vi "DataTransmit.vi"(0 "数据输入":u8[](array[numeric])=array[16384 elements]) -> (2 "输出簇ADC":T4, 4 "输出簇A":T3, 5 "输出簇B":T2, 6 "总输出簇":T1, 7 "总数组":dbl[][](array[numeric]))   [LabVIEW 2014]
uses:
  DataType.ctl
panel:
  out "GlobalAMPValueFPGA":dbl
  out "GlobalAMPValueFPGAB":dbl
  out "GlobalAMPFittingBH2":dbl
  out "GlobalAMPFittingBH1":dbl
  out "GlobalAMPFittingB":dbl
  out "GlobalAMPFittingH2":dbl
  out "GlobalAMPFittingH1":dbl
  out "GlobalAMPFitting":dbl
  out "计数值":u8
  out "AD4":dbl[](array[numeric])
  out "AD3":dbl[](array[numeric])
  out "AD2":dbl[](array[numeric])
  out "AD1":dbl[](array[numeric])
  out "Yh2B":dbl[](array[numeric])
  out "Xh2B":dbl[](array[numeric])
  out "Yh1B":dbl[](array[numeric])
  out "Xh1B":dbl[](array[numeric])
  out "NoiseB":dbl[](array[numeric])
  out "FrequencyB":dbl[](array[numeric])
  out "YB":dbl[](array[numeric])
  out "XB":dbl[](array[numeric])
  out "Yh2A":dbl[](array[numeric])
  out "Xh2A":dbl[](array[numeric])
  out "Yh1A":dbl[](array[numeric])
  out "Xh1A":dbl[](array[numeric])
  out "NoiseA":dbl[](array[numeric])
  out "FrequencyA":dbl[](array[numeric])
  out "YA":dbl[](array[numeric])
  out "XA":dbl[](array[numeric])
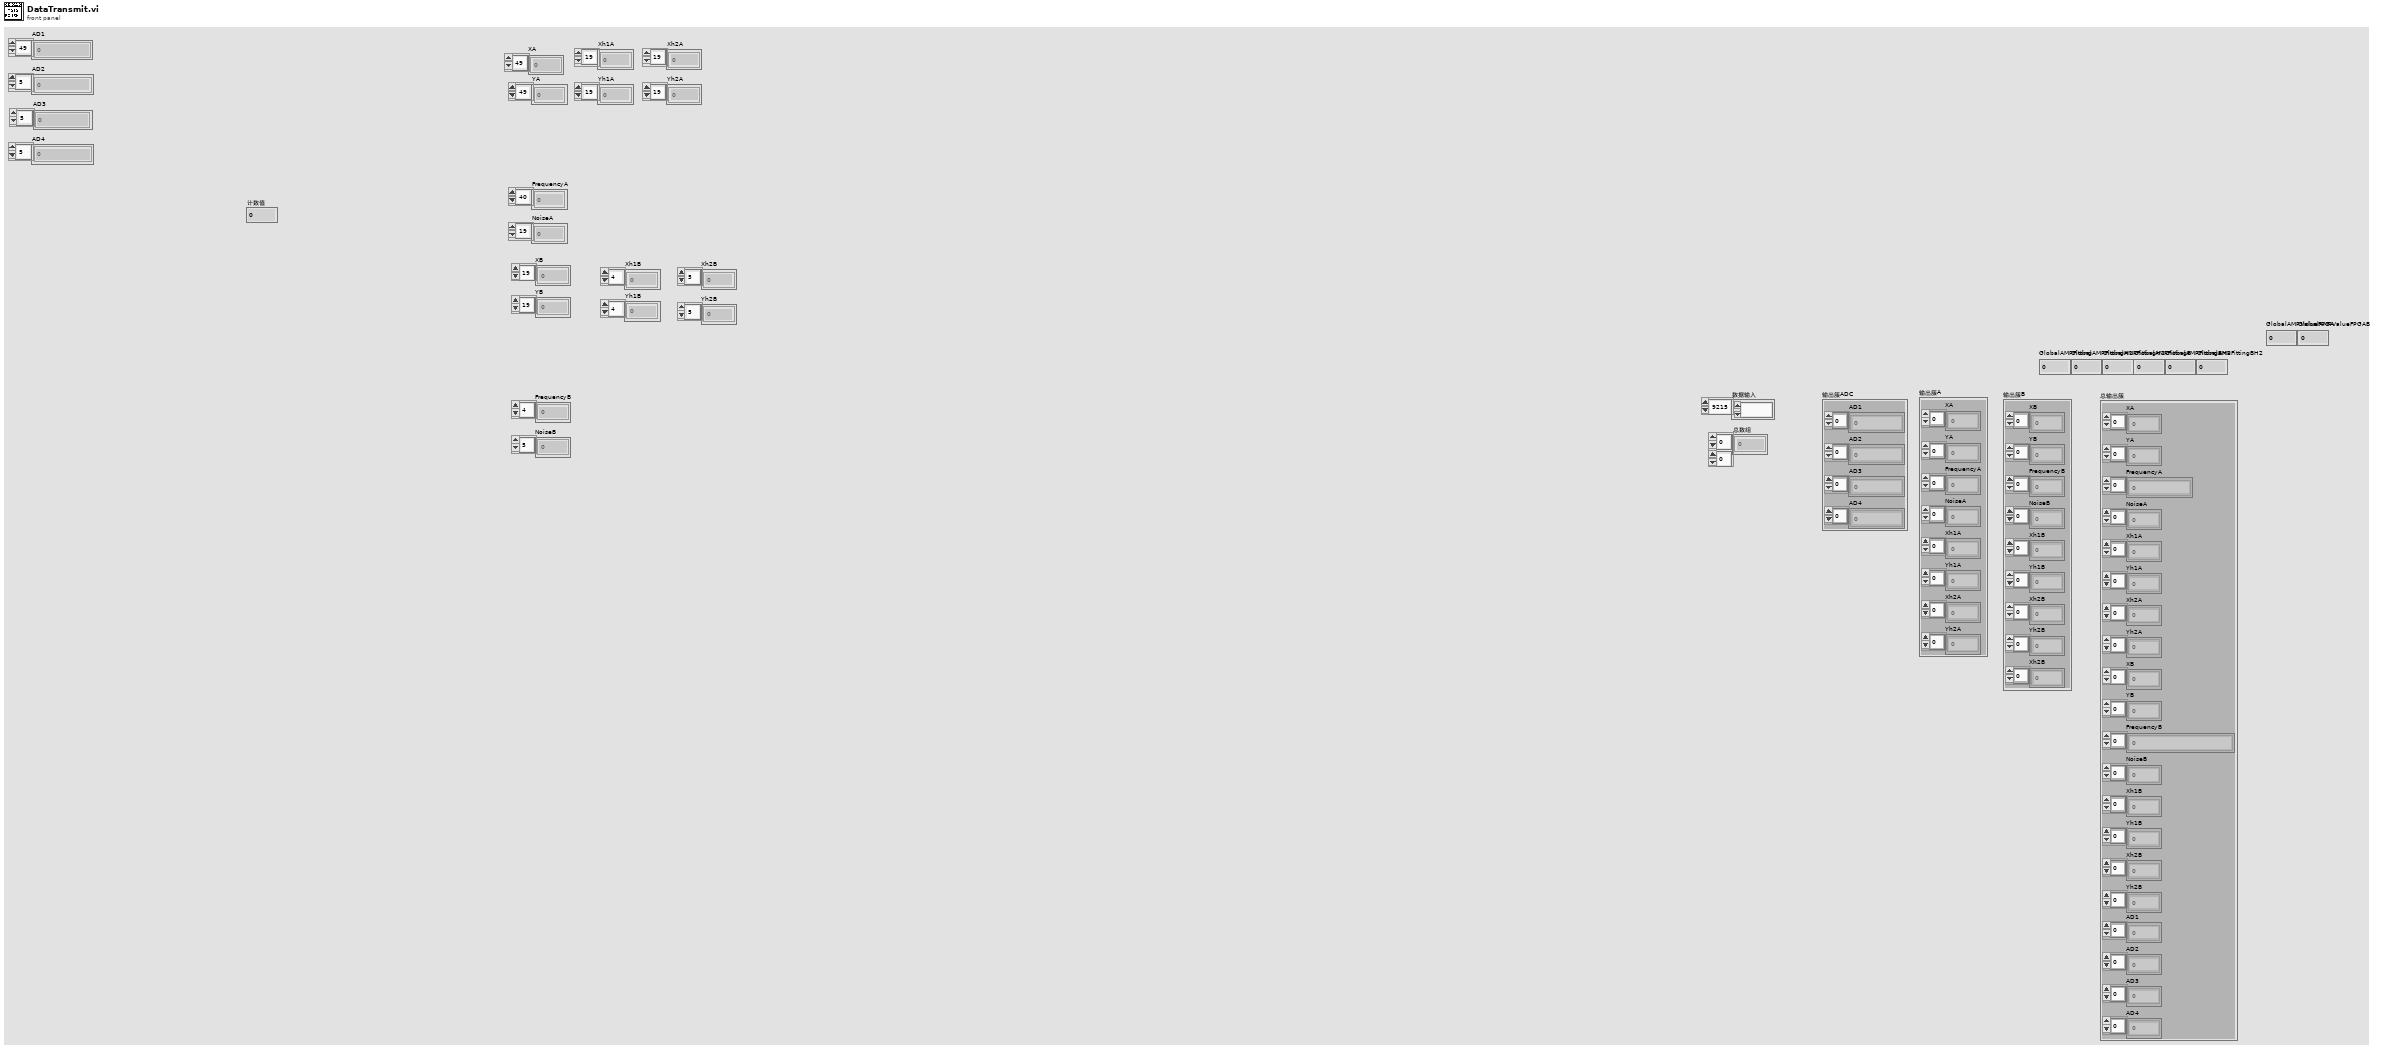
[diagram p1: front panel]
types:
  T1 = cluster{"XA":dbl[], "YA":dbl[], "FrequencyA":dbl[], "NoiseA":dbl[], "Xh1A":dbl[], "Yh1A":dbl[], "Xh2A":dbl[], "Yh2A":dbl[], "XB":dbl[], "YB":dbl[], "FrequencyB":dbl[], "NoiseB":dbl[], "Xh1B":dbl[], "Yh1B":dbl[], "Xh2B":dbl[], "Yh2B":dbl[], "AD1":dbl[], "AD2":dbl[], "AD3":dbl[], "AD4":dbl[]}
  T2 = cluster{"XB":dbl[], "YB":dbl[], "FrequencyB":dbl[], "NoiseB":dbl[], "Xh1B":dbl[], "Yh1B":dbl[], "Xh2B":dbl[], "Yh2B":dbl[], "Xh2B":dbl[]}
  T3 = cluster{"XA":dbl[], "YA":dbl[], "FrequencyA":dbl[], "NoiseA":dbl[], "Xh1A":dbl[], "Yh1A":dbl[], "Xh2A":dbl[], "Yh2A":dbl[]}
  T4 = cluster{"AD1":dbl[], "AD2":dbl[], "AD3":dbl[], "AD4":dbl[]}
  T5 = typedef "DataType.ctl" = u16
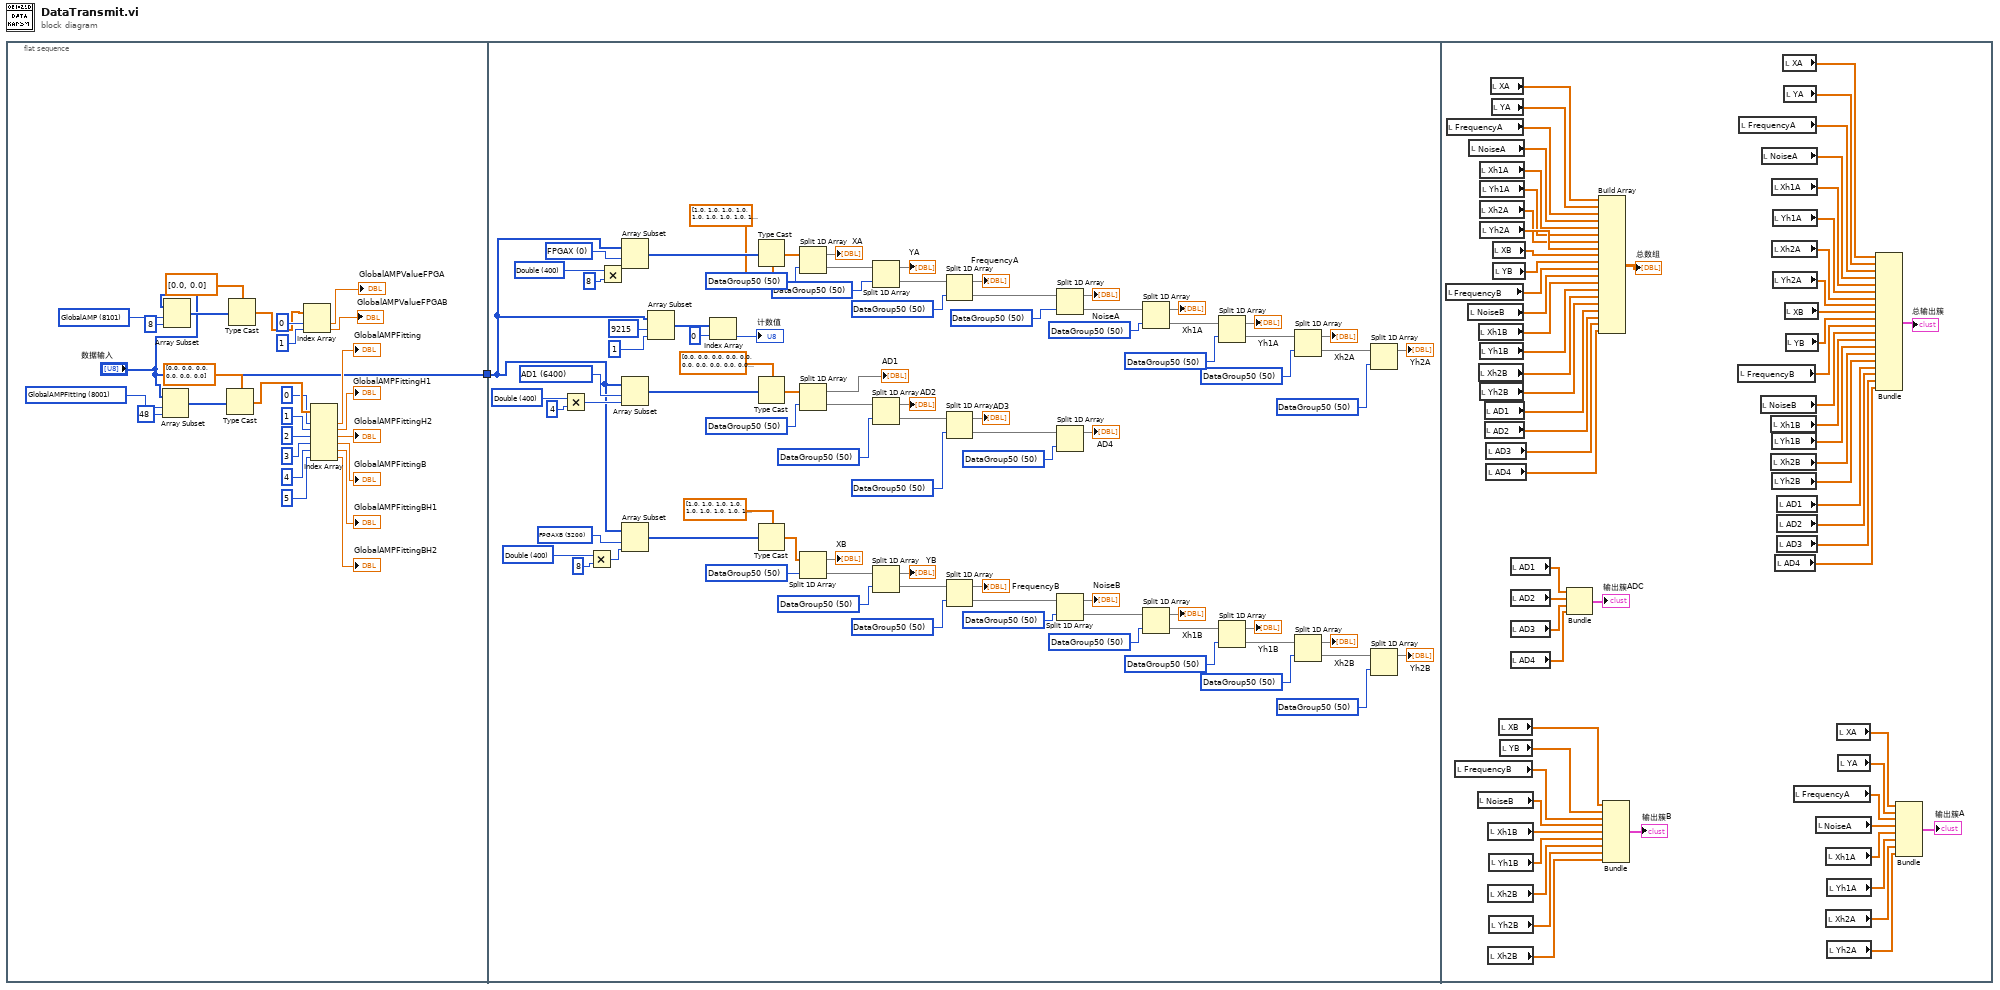
[diagram p0: block diagram]
diagram:
  n1 = flat-sequence {
    tunnel: ["数据输入"] -> w1
    tunnel: w1 -> [w29]
    frame #0 {
      w8 = u32 8101 items=["FPGAX"=0, "FPGAY"=400, "FPGAFreq"=800, "FPGANOISE"=1200, "FPGAXHARM1"=1600, "FPGAYHARM1"=2000, "FPGAXHARM2  "=2400, "FPGAYHARM2  "=2800, "FPGAXB"=3200, "FPGAYB"=3600, "FPGAFreqB"=4000, "FPGANOISEB"=4400, "FPGAXHARM1B"=4800, "FPGAYHARM1B"=5200, "FPGAXHARM2B "=5600, "FPGAYHARM2B "=6000, "AD1           "=6400, "AD2           "=6800, "AD3           "=7200, "AD4   "=7600, "GlobalAMPFitting"=8001, "GlobalAMP"=8101, "FPGAFreq"=7455, "InternalFreqvalue"=7463, "GlobalRefPhaseSlope"=7471, "HarmValue1"=7472, "HarmValue2"=7480, "REFReserve"=7488, "GlobalSweepType"=7496, "InternalSweepSartFreqvalue"=7497, "InternalSweepStopFreqvalue"=7505, "InternalSweepStepFreqvalue"=7513, "InternalSweepStepPercentValue"=7521, "InternalSweepTimeValue"=7525, "GlobalSweepTrigger"=7533, "INTReserve"=7534, "SineOutFixedVoltageValue"=7542, "GlobalSineOutSweepType"=7546, "SineOutSweepStartValue"=7547, "SineOutSweepStopValue"=7551, "SineOutSweepStepValue"=7555, "SineOutSweepStepPercentValue"=7559, "SineOutSweepTimeValue"=7563, "GlobalSineOutSweepTrigger"=7571, "SineReserve"=7572, "EquationC1"=7580, "EquationC2"=7588, "GlobalEquationTypeA"=7596, "GlobalEquationTypeB"=7601, "GlobalEquationTypeC"=7604, "EquatReserve"=7608, "GlobalGainTCSensitivity"=7640, "GlobalGainTCReserve"=7641, "GlobalInputFilterSource"=7642, "GlobalInputFilterGrounding"=7643, "GlobalInputFilterCoupling"=7644, "GlobalInputFilterNotches"=7645, "InputReserve"=7646, "GlobalGainTCTimeConstant"=7654, "GlobalGainTCFliter"=7655, "GlobalGainTCSynchronous"=7656, "FliterReserve"=7657, "GlobalOutputCH1Source"=7665, "GlobalOutputCH2Source"=7666, "Offsetvalue"=7667, "Expandvalue"=7671, "GlobalOutputSpeed"=7673, "GlobalOutputSpeedCH2"=7674, "ChannelReserve"=7675, "SampleStepTimeValue"=7691, "SampleLengthValue"=7699, "Buffer1Source"=7707, "Buffer2Source"=7708, "Buffer3Source"=7709, "Buffer4Source"=7710, "GlobalSampleTriggerMode"=7711, "GlobalSampleRunMode"=7712, "SampleCurrentPoints"=7713, "SampleReserve"=7721, "InputOvldStatusflag"=7729, "GainOvldStatusflag"=7730, "FPGAFreqShift"=7731, "SystemReserve"=7732, "GlobalRefPhasePhaseB"=7800, "GlobalRefPhaseSourceB"=7804, "FPGAFreqB"=7805, "InternalFreqvalueB"=7813, "GlobalRefPhaseSlopeB"=7821, "HarmValue1B"=7822, "HarmValue2B"=7830, "REFReserveB"=7838, "GlobalSweepTypeB"=7846, "InternalSweepSartFreqvalueB"=7847, "InternalSweepStopFreqvalueB"=7855, "InternalSweepStepFreqvalueB"=7863, "InternalSweepStepPercentValueB"=7871, "InternalSweepTimeValueB"=7875, "GlobalSweepTriggerB"=7883, "INTReserveB"=7884, "SineOutFixedVoltageValueB"=7892, "GlobalSineOutSweepTypeB"=7896, "SineOutSweepStartValueB"=7897, "SineOutSweepStopValueB"=7901, "SineOutSweepStepValueB"=7905, "SineOutSweepStepPercentValueB"=7909, "SineOutSweepTimeValueB"=7913, "GlobalSineOutSweepTriggerB"=7921, "SineReserveB"=7922, "EquationC1B"=7930, "EquationC2B"=7938, "GlobalEquationTypeAB"=7946, "GlobalEquationTypeBB"=7950, "GlobalEquationTypeCB"=7954, "EquatReserveB"=7958, "GlobalGainTCSensitivityB"=7990, "GlobalGainTCReserveB"=7991, "GlobalInputFilterSourceB"=7992, "GlobalInputFilterGroundingB"=7993, "GlobalInputFilterCouplingB"=7994, "GlobalInputFilterNotchesB"=7995, "InputReserveB"=7996, "GlobalGainTCTimeConstantB"=8004, "GlobalGainTCFliterB"=8005, "GlobalGainTCSynchronousB"=8006, "FliterReserveB"=8007, "GlobalOutputCH1Source"=8015, "GlobalOutputCH2Source"=8016, "OffsetvalueB"=8017, "ExpandvalueB"=8021, "GlobalOutputSpeedB"=8023, "GlobalOutputSpeedCH2B"=8024, "ChannelReserve"=8025, "SampleStepTimeValueB"=8041, "SampleLengthValueB"=8049, "Buffer1SourceB"=8057, "Buffer2SourceB"=8058, "Buffer3SourceB"=8059, "Buffer4SourceB"=8060, "GlobalSampleTriggerModeB"=8061, "GlobalSampleRunModeB"=8062, "SampleCurrentPointsB"=8063, "SampleReserveB"=8071, "InputOvldStatusflagB"=8079, "GainOvldStatusflagB"=8080, "FPGAFreqShiftB"=8081, "SystemReserveB"=8082] ("下拉列表")
      w28 = u32 8001 items=["FPGAX"=0, "FPGAY"=400, "FPGAFreq"=800, "FPGANOISE"=1200, "FPGAXHARM1"=1600, "FPGAYHARM1"=2000, "FPGAXHARM2  "=2400, "FPGAYHARM2  "=2800, "FPGAXB"=3200, "FPGAYB"=3600, "FPGAFreqB"=4000, "FPGANOISEB"=4400, "FPGAXHARM1B"=4800, "FPGAYHARM1B"=5200, "FPGAXHARM2B "=5600, "FPGAYHARM2B "=6000, "AD1           "=6400, "AD2           "=6800, "AD3           "=7200, "AD4   "=7600, "GlobalAMPFitting"=8001, "GlobalAMP"=8101, "FPGAFreq"=7455, "InternalFreqvalue"=7463, "GlobalRefPhaseSlope"=7471, "HarmValue1"=7472, "HarmValue2"=7480, "REFReserve"=7488, "GlobalSweepType"=7496, "InternalSweepSartFreqvalue"=7497, "InternalSweepStopFreqvalue"=7505, "InternalSweepStepFreqvalue"=7513, "InternalSweepStepPercentValue"=7521, "InternalSweepTimeValue"=7525, "GlobalSweepTrigger"=7533, "INTReserve"=7534, "SineOutFixedVoltageValue"=7542, "GlobalSineOutSweepType"=7546, "SineOutSweepStartValue"=7547, "SineOutSweepStopValue"=7551, "SineOutSweepStepValue"=7555, "SineOutSweepStepPercentValue"=7559, "SineOutSweepTimeValue"=7563, "GlobalSineOutSweepTrigger"=7571, "SineReserve"=7572, "EquationC1"=7580, "EquationC2"=7588, "GlobalEquationTypeA"=7596, "GlobalEquationTypeB"=7601, "GlobalEquationTypeC"=7604, "EquatReserve"=7608, "GlobalGainTCSensitivity"=7640, "GlobalGainTCReserve"=7641, "GlobalInputFilterSource"=7642, "GlobalInputFilterGrounding"=7643, "GlobalInputFilterCoupling"=7644, "GlobalInputFilterNotches"=7645, "InputReserve"=7646, "GlobalGainTCTimeConstant"=7654, "GlobalGainTCFliter"=7655, "GlobalGainTCSynchronous"=7656, "FliterReserve"=7657, "GlobalOutputCH1Source"=7665, "GlobalOutputCH2Source"=7666, "Offsetvalue"=7667, "Expandvalue"=7671, "GlobalOutputSpeed"=7673, "GlobalOutputSpeedCH2"=7674, "ChannelReserve"=7675, "SampleStepTimeValue"=7691, "SampleLengthValue"=7699, "Buffer1Source"=7707, "Buffer2Source"=7708, "Buffer3Source"=7709, "Buffer4Source"=7710, "GlobalSampleTriggerMode"=7711, "GlobalSampleRunMode"=7712, "SampleCurrentPoints"=7713, "SampleReserve"=7721, "InputOvldStatusflag"=7729, "GainOvldStatusflag"=7730, "FPGAFreqShift"=7731, "SystemReserve"=7732, "GlobalRefPhasePhaseB"=7800, "GlobalRefPhaseSourceB"=7804, "FPGAFreqB"=7805, "InternalFreqvalueB"=7813, "GlobalRefPhaseSlopeB"=7821, "HarmValue1B"=7822, "HarmValue2B"=7830, "REFReserveB"=7838, "GlobalSweepTypeB"=7846, "InternalSweepSartFreqvalueB"=7847, "InternalSweepStopFreqvalueB"=7855, "InternalSweepStepFreqvalueB"=7863, "InternalSweepStepPercentValueB"=7871, "InternalSweepTimeValueB"=7875, "GlobalSweepTriggerB"=7883, "INTReserveB"=7884, "SineOutFixedVoltageValueB"=7892, "GlobalSineOutSweepTypeB"=7896, "SineOutSweepStartValueB"=7897, "SineOutSweepStopValueB"=7901, "SineOutSweepStepValueB"=7905, "SineOutSweepStepPercentValueB"=7909, "SineOutSweepTimeValueB"=7913, "GlobalSineOutSweepTriggerB"=7921, "SineReserveB"=7922, "EquationC1B"=7930, "EquationC2B"=7938, "GlobalEquationTypeAB"=7946, "GlobalEquationTypeBB"=7950, "GlobalEquationTypeCB"=7954, "EquatReserveB"=7958, "GlobalGainTCSensitivityB"=7990, "GlobalGainTCReserveB"=7991, "GlobalInputFilterSourceB"=7992, "GlobalInputFilterGroundingB"=7993, "GlobalInputFilterCouplingB"=7994, "GlobalInputFilterNotchesB"=7995, "InputReserveB"=7996, "GlobalGainTCTimeConstantB"=8004, "GlobalGainTCFliterB"=8005, "GlobalGainTCSynchronousB"=8006, "FliterReserveB"=8007, "GlobalOutputCH1Source"=8015, "GlobalOutputCH2Source"=8016, "OffsetvalueB"=8017, "ExpandvalueB"=8021, "GlobalOutputSpeedB"=8023, "GlobalOutputSpeedCH2B"=8024, "ChannelReserve"=8025, "SampleStepTimeValueB"=8041, "SampleLengthValueB"=8049, "Buffer1SourceB"=8057, "Buffer2SourceB"=8058, "Buffer3SourceB"=8059, "Buffer4SourceB"=8060, "GlobalSampleTriggerModeB"=8061, "GlobalSampleRunModeB"=8062, "SampleCurrentPointsB"=8063, "SampleReserveB"=8071, "InputOvldStatusflagB"=8079, "GainOvldStatusflagB"=8080, "FPGAFreqShiftB"=8081, "SystemReserveB"=8082] ("下拉列表")
      n2 = Array Subset(array="数据输入", index=w28, length=48 ("长度")) -> (w25:u8[])
      n3 = Array Subset(array="数据输入", index=w8, length=8 ("长度")) -> (w11:u8[])
      n4 = Type Cast(type=dbl[] [0.0, 0.0, 0.0, 0.0, 0.0, 0.0], x=w25) -> (*(type *) &x=w24:dbl[])
      n5 = Type Cast(type=sgl[] [0.0, 0.0], x=w11) -> (*(type *) &x=w2:sgl[])
      n6 = Index Array(array=w2, index #1=0 ("索引"), index #2=1 ("索引 2")) -> (element #1=→"GlobalAMPValueFPGA":sgl, element #2=→"GlobalAMPValueFPGAB":sgl)
      n7 = Index Array(array=w24, index #1=0 ("索引"), index #2=1 ("索引 2"), index #3=2 ("索引 3"), index #4=3 ("索引 4"), index #5=4 ("索引 5"), index #6=5 ("索引 6")) -> (element #1=→"GlobalAMPFitting":dbl, element #2=→"GlobalAMPFittingH1":dbl, element #3=→"GlobalAMPFittingH2":dbl, element #4=→"GlobalAMPFittingB":dbl, element #5=→"GlobalAMPFittingBH1":dbl, element #6=→"GlobalAMPFittingBH2":dbl)
    }
    frame #1 {
      w112 = u16 50 items=["unsignedInt8"=1, "unsignedInt16"=2, "unsignedInt32"=4, "unsignedInt64"=8, "Float"=80, "Double"=160, "StartLength"=2240, "DataGroup50"=50, "DataGroup20"=20] ("数据类型")
      w111 = u16 50 items=["unsignedInt8"=1, "unsignedInt16"=2, "unsignedInt32"=4, "unsignedInt64"=8, "Float"=80, "Double"=160, "StartLength"=2240, "DataGroup50"=50, "DataGroup20"=20] ("数据类型")
      w109 = u16 50 items=["unsignedInt8"=1, "unsignedInt16"=2, "unsignedInt32"=4, "unsignedInt64"=8, "Float"=80, "Double"=160, "StartLength"=2240, "DataGroup50"=50, "DataGroup20"=20] ("数据类型")
      w108 = u16 50 items=["unsignedInt8"=1, "unsignedInt16"=2, "unsignedInt32"=4, "unsignedInt64"=8, "Float"=80, "Double"=160, "StartLength"=2240, "DataGroup50"=50, "DataGroup20"=20] ("数据类型")
      w107 = u16 50 items=["unsignedInt8"=1, "unsignedInt16"=2, "unsignedInt32"=4, "unsignedInt64"=8, "Float"=80, "Double"=160, "StartLength"=2240, "DataGroup50"=50, "DataGroup20"=20] ("数据类型")
      w106 = u16 50 items=["unsignedInt8"=1, "unsignedInt16"=2, "unsignedInt32"=4, "unsignedInt64"=8, "Float"=80, "Double"=160, "StartLength"=2240, "DataGroup50"=50, "DataGroup20"=20] ("数据类型")
      w105 = u16 50 items=["unsignedInt8"=1, "unsignedInt16"=2, "unsignedInt32"=4, "unsignedInt64"=8, "Float"=80, "Double"=160, "StartLength"=2240, "DataGroup50"=50, "DataGroup20"=20] ("数据类型")
      w110 = u16 50 items=["unsignedInt8"=1, "unsignedInt16"=2, "unsignedInt32"=4, "unsignedInt64"=8, "Float"=80, "Double"=160, "StartLength"=2240, "DataGroup50"=50, "DataGroup20"=20] ("数据类型")
      w104 = u16 50 items=["unsignedInt8"=1, "unsignedInt16"=2, "unsignedInt32"=4, "unsignedInt64"=8, "Float"=80, "Double"=160, "StartLength"=2240, "DataGroup50"=50, "DataGroup20"=20] ("数据类型")
      w103 = u16 50 items=["unsignedInt8"=1, "unsignedInt16"=2, "unsignedInt32"=4, "unsignedInt64"=8, "Float"=80, "Double"=160, "StartLength"=2240, "DataGroup50"=50, "DataGroup20"=20] ("数据类型")
      w96 = T5 400 items=["unsignedInt8"=1, "unsignedInt16"=2, "unsignedInt32"=4, "unsignedInt64"=8, "Float"=200, "Double"=400] ("数据类型")
      w95 = u32 3200 items=["FPGAX"=0, "FPGAY"=400, "FPGAFreq"=800, "FPGANOISE"=1200, "FPGAXHARM1"=1600, "FPGAYHARM1"=2000, "FPGAXHARM2  "=2400, "FPGAYHARM2  "=2800, "FPGAXB"=3200, "FPGAYB"=3600, "FPGAFreqB"=4000, "FPGANOISEB"=4400, "FPGAXHARM1B"=4800, "FPGAYHARM1B"=5200, "FPGAXHARM2B "=5600, "FPGAYHARM2B "=6000, "AD1           "=6400, "AD2           "=6800, "AD3           "=7200, "AD4   "=7600, "GlobalRefPhasePhase"=7450, "GlobalRefPhaseSource"=7454, "FPGAFreq"=7455, "InternalFreqvalue"=7463, "GlobalRefPhaseSlope"=7471, "HarmValue1"=7472, "HarmValue2"=7480, "REFReserve"=7488, "GlobalSweepType"=7496, "InternalSweepSartFreqvalue"=7497, "InternalSweepStopFreqvalue"=7505, "InternalSweepStepFreqvalue"=7513, "InternalSweepStepPercentValue"=7521, "InternalSweepTimeValue"=7525, "GlobalSweepTrigger"=7533, "INTReserve"=7534, "SineOutFixedVoltageValue"=7542, "GlobalSineOutSweepType"=7546, "SineOutSweepStartValue"=7547, "SineOutSweepStopValue"=7551, "SineOutSweepStepValue"=7555, "SineOutSweepStepPercentValue"=7559, "SineOutSweepTimeValue"=7563, "GlobalSineOutSweepTrigger"=7571, "SineReserve"=7572, "EquationC1"=7580, "EquationC2"=7588, "GlobalEquationTypeA"=7596, "GlobalEquationTypeB"=7601, "GlobalEquationTypeC"=7604, "EquatReserve"=7608, "GlobalGainTCSensitivity"=7640, "GlobalGainTCReserve"=7641, "GlobalInputFilterSource"=7642, "GlobalInputFilterGrounding"=7643, "GlobalInputFilterCoupling"=7644, "GlobalInputFilterNotches"=7645, "InputReserve"=7646, "GlobalGainTCTimeConstant"=7654, "GlobalGainTCFliter"=7655, "GlobalGainTCSynchronous"=7656, "FliterReserve"=7657, "GlobalOutputCH1Source"=7665, "GlobalOutputCH2Source"=7666, "Offsetvalue"=7667, "Expandvalue"=7671, "GlobalOutputSpeed"=7673, "GlobalOutputSpeedCH2"=7674, "ChannelReserve"=7675, "SampleStepTimeValue"=7691, "SampleLengthValue"=7699, "Buffer1Source"=7707, "Buffer2Source"=7708, "Buffer3Source"=7709, "Buffer4Source"=7710, "GlobalSampleTriggerMode"=7711, "GlobalSampleRunMode"=7712, "SampleCurrentPoints"=7713, "SampleReserve"=7721, "InputOvldStatusflag"=7729, "GainOvldStatusflag"=7730, "FPGAFreqShift"=7731, "SystemReserve"=7732, "GlobalRefPhasePhaseB"=7800, "GlobalRefPhaseSourceB"=7804, "FPGAFreqB"=7805, "InternalFreqvalueB"=7813, "GlobalRefPhaseSlopeB"=7821, "HarmValue1B"=7822, "HarmValue2B"=7830, "REFReserveB"=7838, "GlobalSweepTypeB"=7846, "InternalSweepSartFreqvalueB"=7847, "InternalSweepStopFreqvalueB"=7855, "InternalSweepStepFreqvalueB"=7863, "InternalSweepStepPercentValueB"=7871, "InternalSweepTimeValueB"=7875, "GlobalSweepTriggerB"=7883, "INTReserveB"=7884, "SineOutFixedVoltageValueB"=7892, "GlobalSineOutSweepTypeB"=7896, "SineOutSweepStartValueB"=7897, "SineOutSweepStopValueB"=7901, "SineOutSweepStepValueB"=7905, "SineOutSweepStepPercentValueB"=7909, "SineOutSweepTimeValueB"=7913, "GlobalSineOutSweepTriggerB"=7921, "SineReserveB"=7922, "EquationC1B"=7930, "EquationC2B"=7938, "GlobalEquationTypeAB"=7946, "GlobalEquationTypeBB"=7950, "GlobalEquationTypeCB"=7954, "EquatReserveB"=7958, "GlobalGainTCSensitivityB"=7990, "GlobalGainTCReserveB"=7991, "GlobalInputFilterSourceB"=7992, "GlobalInputFilterGroundingB"=7993, "GlobalInputFilterCouplingB"=7994, "GlobalInputFilterNotchesB"=7995, "InputReserveB"=7996, "GlobalGainTCTimeConstantB"=8004, "GlobalGainTCFliterB"=8005, "GlobalGainTCSynchronousB"=8006, "FliterReserveB"=8007, "GlobalOutputCH1Source"=8015, "GlobalOutputCH2Source"=8016, "OffsetvalueB"=8017, "ExpandvalueB"=8021, "GlobalOutputSpeedB"=8023, "GlobalOutputSpeedCH2B"=8024, "ChannelReserve"=8025, "SampleStepTimeValueB"=8041, "SampleLengthValueB"=8049, "Buffer1SourceB"=8057, "Buffer2SourceB"=8058, "Buffer3SourceB"=8059, "Buffer4SourceB"=8060, "GlobalSampleTriggerModeB"=8061, "GlobalSampleRunModeB"=8062, "SampleCurrentPointsB"=8063, "SampleReserveB"=8071, "InputOvldStatusflagB"=8079, "GainOvldStatusflagB"=8080, "FPGAFreqShiftB"=8081, "SystemReserveB"=8082] ("下拉列表")
      w94 = u16 50 items=["unsignedInt8"=1, "unsignedInt16"=2, "unsignedInt32"=4, "unsignedInt64"=8, "Float"=80, "Double"=160, "StartLength"=2240, "DataGroup50"=50, "DataGroup20"=20] ("数据类型")
      w93 = u16 50 items=["unsignedInt8"=1, "unsignedInt16"=2, "unsignedInt32"=4, "unsignedInt64"=8, "Float"=80, "Double"=160, "StartLength"=2240, "DataGroup50"=50, "DataGroup20"=20] ("数据类型")
      w92 = u16 50 items=["unsignedInt8"=1, "unsignedInt16"=2, "unsignedInt32"=4, "unsignedInt64"=8, "Float"=80, "Double"=160, "StartLength"=2240, "DataGroup50"=50, "DataGroup20"=20] ("数据类型")
      w91 = u16 50 items=["unsignedInt8"=1, "unsignedInt16"=2, "unsignedInt32"=4, "unsignedInt64"=8, "Float"=80, "Double"=160, "StartLength"=2240, "DataGroup50"=50, "DataGroup20"=20] ("数据类型")
      w88 = u16 50 items=["unsignedInt8"=1, "unsignedInt16"=2, "unsignedInt32"=4, "unsignedInt64"=8, "Float"=80, "Double"=160, "StartLength"=2240, "DataGroup50"=50, "DataGroup20"=20] ("数据类型")
      w87 = u16 50 items=["unsignedInt8"=1, "unsignedInt16"=2, "unsignedInt32"=4, "unsignedInt64"=8, "Float"=80, "Double"=160, "StartLength"=2240, "DataGroup50"=50, "DataGroup20"=20] ("数据类型")
      w84 = T5 400 items=["unsignedInt8"=1, "unsignedInt16"=2, "unsignedInt32"=4, "unsignedInt64"=8, "Float"=200, "Double"=400] ("数据类型")
      w83 = u32 0 items=["FPGAX"=0, "FPGAY"=400, "FPGAFreq"=800, "FPGANOISE"=1200, "FPGAXHARM1"=1600, "FPGAYHARM1"=2000, "FPGAXHARM2  "=2400, "FPGAYHARM2  "=2800, "FPGAXB"=3200, "FPGAYB"=3600, "FPGAFreqB"=4000, "FPGANOISEB"=4400, "FPGAXHARM1B"=4800, "FPGAYHARM1B"=5200, "FPGAXHARM2B "=5600, "FPGAYHARM2B "=6000, "AD1           "=6400, "AD2           "=6800, "AD3           "=7200, "AD4   "=7600, "GlobalRefPhasePhase"=7450, "GlobalRefPhaseSource"=7454, "FPGAFreq"=7455, "InternalFreqvalue"=7463, "GlobalRefPhaseSlope"=7471, "HarmValue1"=7472, "HarmValue2"=7480, "REFReserve"=7488, "GlobalSweepType"=7496, "InternalSweepSartFreqvalue"=7497, "InternalSweepStopFreqvalue"=7505, "InternalSweepStepFreqvalue"=7513, "InternalSweepStepPercentValue"=7521, "InternalSweepTimeValue"=7525, "GlobalSweepTrigger"=7533, "INTReserve"=7534, "SineOutFixedVoltageValue"=7542, "GlobalSineOutSweepType"=7546, "SineOutSweepStartValue"=7547, "SineOutSweepStopValue"=7551, "SineOutSweepStepValue"=7555, "SineOutSweepStepPercentValue"=7559, "SineOutSweepTimeValue"=7563, "GlobalSineOutSweepTrigger"=7571, "SineReserve"=7572, "EquationC1"=7580, "EquationC2"=7588, "GlobalEquationTypeA"=7596, "GlobalEquationTypeB"=7601, "GlobalEquationTypeC"=7604, "EquatReserve"=7608, "GlobalGainTCSensitivity"=7640, "GlobalGainTCReserve"=7641, "GlobalInputFilterSource"=7642, "GlobalInputFilterGrounding"=7643, "GlobalInputFilterCoupling"=7644, "GlobalInputFilterNotches"=7645, "InputReserve"=7646, "GlobalGainTCTimeConstant"=7654, "GlobalGainTCFliter"=7655, "GlobalGainTCSynchronous"=7656, "FliterReserve"=7657, "GlobalOutputCH1Source"=7665, "GlobalOutputCH2Source"=7666, "Offsetvalue"=7667, "Expandvalue"=7671, "GlobalOutputSpeed"=7673, "GlobalOutputSpeedCH2"=7674, "ChannelReserve"=7675, "SampleStepTimeValue"=7691, "SampleLengthValue"=7699, "Buffer1Source"=7707, "Buffer2Source"=7708, "Buffer3Source"=7709, "Buffer4Source"=7710, "GlobalSampleTriggerMode"=7711, "GlobalSampleRunMode"=7712, "SampleCurrentPoints"=7713, "SampleReserve"=7721, "InputOvldStatusflag"=7729, "GainOvldStatusflag"=7730, "FPGAFreqShift"=7731, "SystemReserve"=7732, "GlobalRefPhasePhaseB"=7800, "GlobalRefPhaseSourceB"=7804, "FPGAFreqB"=7805, "InternalFreqvalueB"=7813, "GlobalRefPhaseSlopeB"=7821, "HarmValue1B"=7822, "HarmValue2B"=7830, "REFReserveB"=7838, "GlobalSweepTypeB"=7846, "InternalSweepSartFreqvalueB"=7847, "InternalSweepStopFreqvalueB"=7855, "InternalSweepStepFreqvalueB"=7863, "InternalSweepStepPercentValueB"=7871, "InternalSweepTimeValueB"=7875, "GlobalSweepTriggerB"=7883, "INTReserveB"=7884, "SineOutFixedVoltageValueB"=7892, "GlobalSineOutSweepTypeB"=7896, "SineOutSweepStartValueB"=7897, "SineOutSweepStopValueB"=7901, "SineOutSweepStepValueB"=7905, "SineOutSweepStepPercentValueB"=7909, "SineOutSweepTimeValueB"=7913, "GlobalSineOutSweepTriggerB"=7921, "SineReserveB"=7922, "EquationC1B"=7930, "EquationC2B"=7938, "GlobalEquationTypeAB"=7946, "GlobalEquationTypeBB"=7950, "GlobalEquationTypeCB"=7954, "EquatReserveB"=7958, "GlobalGainTCSensitivityB"=7990, "GlobalGainTCReserveB"=7991, "GlobalInputFilterSourceB"=7992, "GlobalInputFilterGroundingB"=7993, "GlobalInputFilterCouplingB"=7994, "GlobalInputFilterNotchesB"=7995, "InputReserveB"=7996, "GlobalGainTCTimeConstantB"=8004, "GlobalGainTCFliterB"=8005, "GlobalGainTCSynchronousB"=8006, "FliterReserveB"=8007, "GlobalOutputCH1Source"=8015, "GlobalOutputCH2Source"=8016, "OffsetvalueB"=8017, "ExpandvalueB"=8021, "GlobalOutputSpeedB"=8023, "GlobalOutputSpeedCH2B"=8024, "ChannelReserve"=8025, "SampleStepTimeValueB"=8041, "SampleLengthValueB"=8049, "Buffer1SourceB"=8057, "Buffer2SourceB"=8058, "Buffer3SourceB"=8059, "Buffer4SourceB"=8060, "GlobalSampleTriggerModeB"=8061, "GlobalSampleRunModeB"=8062, "SampleCurrentPointsB"=8063, "SampleReserveB"=8071, "InputOvldStatusflagB"=8079, "GainOvldStatusflagB"=8080, "FPGAFreqShiftB"=8081, "SystemReserveB"=8082] ("下拉列表")
      w82 = u16 50 items=["unsignedInt8"=1, "unsignedInt16"=2, "unsignedInt32"=4, "unsignedInt64"=8, "Float"=80, "Double"=160, "StartLength"=2240, "DataGroup50"=50, "DataGroup20"=20] ("数据类型")
      w81 = u16 50 items=["unsignedInt8"=1, "unsignedInt16"=2, "unsignedInt32"=4, "unsignedInt64"=8, "Float"=80, "Double"=160, "StartLength"=2240, "DataGroup50"=50, "DataGroup20"=20] ("数据类型")
      w80 = u16 50 items=["unsignedInt8"=1, "unsignedInt16"=2, "unsignedInt32"=4, "unsignedInt64"=8, "Float"=80, "Double"=160, "StartLength"=2240, "DataGroup50"=50, "DataGroup20"=20] ("数据类型")
      w78 = u32 6400 items=["FPGAX"=0, "FPGAY"=400, "FPGAFreq"=800, "FPGANOISE"=1200, "FPGAXHARM1"=1600, "FPGAYHARM1"=2000, "FPGAXHARM2  "=2400, "FPGAYHARM2  "=2800, "FPGAXB"=3200, "FPGAYB"=3600, "FPGAFreqB"=4000, "FPGANOISEB"=4400, "FPGAXHARM1B"=4800, "FPGAYHARM1B"=5200, "FPGAXHARM2B "=5600, "FPGAYHARM2B "=6000, "AD1           "=6400, "AD2           "=6800, "AD3           "=7200, "AD4   "=7600, "GlobalRefPhasePhase"=7450, "GlobalRefPhaseSource"=7454, "FPGAFreq"=7455, "InternalFreqvalue"=7463, "GlobalRefPhaseSlope"=7471, "HarmValue1"=7472, "HarmValue2"=7480, "REFReserve"=7488, "GlobalSweepType"=7496, "InternalSweepSartFreqvalue"=7497, "InternalSweepStopFreqvalue"=7505, "InternalSweepStepFreqvalue"=7513, "InternalSweepStepPercentValue"=7521, "InternalSweepTimeValue"=7525, "GlobalSweepTrigger"=7533, "INTReserve"=7534, "SineOutFixedVoltageValue"=7542, "GlobalSineOutSweepType"=7546, "SineOutSweepStartValue"=7547, "SineOutSweepStopValue"=7551, "SineOutSweepStepValue"=7555, "SineOutSweepStepPercentValue"=7559, "SineOutSweepTimeValue"=7563, "GlobalSineOutSweepTrigger"=7571, "SineReserve"=7572, "EquationC1"=7580, "EquationC2"=7588, "GlobalEquationTypeA"=7596, "GlobalEquationTypeB"=7601, "GlobalEquationTypeC"=7604, "EquatReserve"=7608, "GlobalGainTCSensitivity"=7640, "GlobalGainTCReserve"=7641, "GlobalInputFilterSource"=7642, "GlobalInputFilterGrounding"=7643, "GlobalInputFilterCoupling"=7644, "GlobalInputFilterNotches"=7645, "InputReserve"=7646, "GlobalGainTCTimeConstant"=7654, "GlobalGainTCFliter"=7655, "GlobalGainTCSynchronous"=7656, "FliterReserve"=7657, "GlobalOutputCH1Source"=7665, "GlobalOutputCH2Source"=7666, "Offsetvalue"=7667, "Expandvalue"=7671, "GlobalOutputSpeed"=7673, "GlobalOutputSpeedCH2"=7674, "ChannelReserve"=7675, "SampleStepTimeValue"=7691, "SampleLengthValue"=7699, "Buffer1Source"=7707, "Buffer2Source"=7708, "Buffer3Source"=7709, "Buffer4Source"=7710, "GlobalSampleTriggerMode"=7711, "GlobalSampleRunMode"=7712, "SampleCurrentPoints"=7713, "SampleReserve"=7721, "InputOvldStatusflag"=7729, "GainOvldStatusflag"=7730, "FPGAFreqShift"=7731, "SystemReserve"=7732, "GlobalRefPhasePhaseB"=7800, "GlobalRefPhaseSourceB"=7804, "FPGAFreqB"=7805, "InternalFreqvalueB"=7813, "GlobalRefPhaseSlopeB"=7821, "HarmValue1B"=7822, "HarmValue2B"=7830, "REFReserveB"=7838, "GlobalSweepTypeB"=7846, "InternalSweepSartFreqvalueB"=7847, "InternalSweepStopFreqvalueB"=7855, "InternalSweepStepFreqvalueB"=7863, "InternalSweepStepPercentValueB"=7871, "InternalSweepTimeValueB"=7875, "GlobalSweepTriggerB"=7883, "INTReserveB"=7884, "SineOutFixedVoltageValueB"=7892, "GlobalSineOutSweepTypeB"=7896, "SineOutSweepStartValueB"=7897, "SineOutSweepStopValueB"=7901, "SineOutSweepStepValueB"=7905, "SineOutSweepStepPercentValueB"=7909, "SineOutSweepTimeValueB"=7913, "GlobalSineOutSweepTriggerB"=7921, "SineReserveB"=7922, "EquationC1B"=7930, "EquationC2B"=7938, "GlobalEquationTypeAB"=7946, "GlobalEquationTypeBB"=7950, "GlobalEquationTypeCB"=7954, "EquatReserveB"=7958, "GlobalGainTCSensitivityB"=7990, "GlobalGainTCReserveB"=7991, "GlobalInputFilterSourceB"=7992, "GlobalInputFilterGroundingB"=7993, "GlobalInputFilterCouplingB"=7994, "GlobalInputFilterNotchesB"=7995, "InputReserveB"=7996, "GlobalGainTCTimeConstantB"=8004, "GlobalGainTCFliterB"=8005, "GlobalGainTCSynchronousB"=8006, "FliterReserveB"=8007, "GlobalOutputCH1Source"=8015, "GlobalOutputCH2Source"=8016, "OffsetvalueB"=8017, "ExpandvalueB"=8021, "GlobalOutputSpeedB"=8023, "GlobalOutputSpeedCH2B"=8024, "ChannelReserve"=8025, "SampleStepTimeValueB"=8041, "SampleLengthValueB"=8049, "Buffer1SourceB"=8057, "Buffer2SourceB"=8058, "Buffer3SourceB"=8059, "Buffer4SourceB"=8060, "GlobalSampleTriggerModeB"=8061, "GlobalSampleRunModeB"=8062, "SampleCurrentPointsB"=8063, "SampleReserveB"=8071, "InputOvldStatusflagB"=8079, "GainOvldStatusflagB"=8080, "FPGAFreqShiftB"=8081, "SystemReserveB"=8082] ("下拉列表")
      w62 = u16 50 items=["unsignedInt8"=1, "unsignedInt16"=2, "unsignedInt32"=4, "unsignedInt64"=8, "Float"=80, "Double"=160, "StartLength"=2240, "DataGroup50"=50, "DataGroup20"=20] ("数据类型")
      w31 = T5 400 items=["unsignedInt8"=1, "unsignedInt16"=2, "unsignedInt32"=4, "unsignedInt64"=8, "Float"=80, "Double"=400] ("数据类型")
      n8 = Multiply(x=w31, y=4) -> (x*y=w68:i32)
      n9 = Multiply(x=w96, y=8) -> (x*y=w97:i32)
      n10 = Multiply(x=w84, y=8) -> (x*y=w85:i32)
      n11 = Array Subset(array=w29, index=w83, length=w85) -> (w70:u8[])
      n12 = Array Subset(array=w29, index=w78, length=w68) -> (w72:u8[])
      n13 = Array Subset(array=w29, index=w95, length=w97) -> (w71:u8[])
      n14 = Array Subset(array=w29, index=9215 ("索引"), length=1 ("索引")) -> (w75:u8[])
      n15 = Index Array(array=w75, index=0 ("索引")) -> (element=→"计数值":u8)
      n16 = Type Cast(type=dbl[] [1.0, 1.0, 1.0, 1.0, 1.0, 1.0, 1.0, 1.0, 1.0, 1.0, 1.0, 1.0, 1.0, 1.0, 1.0, 1.0, 1.0, 1.0, 1.0, 1.0, 1.0, 1.0, 1.0, 1.0, 1.0, 1.0, 1.0, 1.0, 1.0, 1.0, 1.0, 1.0, 1.0, 1.0, 1.0, 1.0, 1.0, 1.0, 1.0, 1.0, 1.0, 1.0, 1.0, 1.0, 1.0, 1.0, 1.0, 1.0, 1.0, 1.0, 1.0, 1.0, 1.0, 1.0, 1.0, 1.0, 1.0, 1.0, 1.0, 1.0, 1.0, 1.0, 1.0, 1.0, 1.0, 1.0, 1.0, 1.0, 1.0, 1.0, 1.0, 1.0, 1.0, 1.0, 1.0, 1.0, 1.0, 1.0, 1.0, 1.0, 1.0, 1.0, 1.0, 1.0, 1.0, 1.0, 1.0, 1.0, 1.0, 1.0, 1.0, 1.0, 1.0, 1.0, 1.0, 1.0, 1.0, 1.0, 1.0, 1.0, 1.0, 1.0, 1.0, 1.0, 1.0, 1.0, 1.0, 1.0, 1.0, 1.0, 1.0, 1.0, 1.0, 1.0, 1.0, 1.0, 1.0, 1.0, 1.0, 1.0, 1.0, 1.0, 1.0, 1.0, 1.0, 1.0, 1.0, 1.0, 1.0, 1.0, 1.0, 1.0, 1.0, 1.0, 1.0, 1.0, 1.0, 1.0, 1.0, 1.0, 1.0, 1.0, 1.0, 1.0, 1.0, 1.0, 1.0, 1.0, 1.0, 1.0, 1.0, 1.0, 1.0, 1.0, 1.0, 1.0, 1.0, 1.0, 1.0, 1.0, 1.0, 1.0, 1.0, 1.0, 1.0, 1.0, 1.0, 1.0, 1.0, 1.0, 1.0, 1.0, 1.0, 1.0, 1.0, 1.0, 1.0, 1.0, 1.0, 1.0, 1.0, 1.0, 1.0, 1.0, 1.0, 1.0, 1.0, 1.0, 1.0, 1.0, 1.0, 1.0, 1.0, 1.0, 1.0, 1.0, 1.0, 1.0, 1.0, 1.0, 1.0, 1.0, 1.0, 1.0, 1.0, 1.0, 1.0, 1.0, 1.0, 1.0, 1.0, 1.0, 1.0, 1.0, 1.0, 1.0, 1.0, 1.0, 1.0, 1.0, 1.0, 1.0, 1.0, 1.0, 1.0, 1.0, 1.0, 1.0, 1.0, 1.0, 1.0, 1.0, 1.0, 1.0, 1.0, 1.0, 1.0, 1.0, 1.0, 1.0, 1.0, 1.0, 1.0, 1.0, 1.0, 1.0, 1.0, 1.0, 1.0, 1.0, 1.0, 1.0, 1.0, 1.0, 1.0, 1.0, 1.0, 1.0, 1.0, 1.0, 1.0, 1.0, 1.0, 1.0, 1.0, 1.0, 1.0, 1.0, 1.0, 1.0, 1.0, 1.0, 1.0, 1.0, 1.0, 1.0, 1.0, 1.0, 1.0, 1.0, 1.0, 1.0, 1.0, 1.0, 1.0, 1.0, 1.0, 1.0, 1.0, 1.0, 1.0, 1.0, 1.0, 1.0, 1.0, 1.0, 1.0, 1.0, 1.0, 1.0, 1.0, 1.0, 1.0, 1.0, 1.0, 1.0, 1.0, 1.0, 1.0, 1.0, 1.0, 1.0, 1.0, 1.0, 1.0, 1.0, 1.0, 1.0, 1.0, 1.0, 1.0, 1.0, 1.0, 1.0, 1.0, 1.0, 1.0, 1.0, 1.0, 1.0, 1.0, 1.0, 1.0, 1.0, 1.0, 1.0, 1.0, 1.0, 1.0, 1.0, 1.0, 1.0, 1.0, 1.0, 1.0, 1.0, 1.0, 1.0, 1.0, 1.0, 1.0, 1.0, 1.0, 1.0, 1.0, 1.0, 1.0, 1.0, 1.0, 1.0, 1.0, 1.0, 1.0, 1.0, 1.0, 1.0, 1.0, 1.0, 1.0, 1.0, 1.0, 1.0, 1.0, 1.0, 1.0, 1.0, 1.0, 1.0, 1.0, 1.0, 1.0, 1.0, 1.0, 1.0, 1.0, 1.0, 1.0, 1.0, 1.0, 1.0, 1.0, 1.0, 1.0, 1.0, 1.0, 1.0, 1.0, 1.0, 1.0, 1.0], x=w70) -> (*(type *) &x=w33:dbl[])
      n17 = Type Cast(type=dbl[] [0.0, 0.0, 0.0, 0.0, 0.0, 0.0, 0.0, 0.0, 0.0, 0.0, 0.0, 0.0, 0.0, 0.0, 0.0, 0.0, 0.0, 0.0, 0.0, 1.0, 0.0, 0.0, 0.0, 0.0, 0.0, 0.0, 0.0, 0.0, 0.0, 0.0, 0.0, 0.0, 0.0, 0.0, 0.0, 0.0, 0.0, 0.0, 0.0, 0.0, 0.0, 0.0, 0.0, 0.0, 0.0, 0.0, 0.0, 0.0, 0.0, 0.0, 0.0, 0.0, 0.0, 0.0, 0.0, 0.0, 0.0, 0.0, 0.0, 0.0, 0.0, 0.0, 0.0, 0.0, 0.0, 0.0, 0.0, 0.0, 0.0, 0.0, 0.0, 0.0, 0.0, 0.0, 0.0, 0.0, 0.0, 0.0, 0.0, 1.0, 0.0, 0.0, 0.0, 0.0, 0.0, 0.0, 0.0, 0.0, 0.0, 0.0, 0.0, 0.0, 0.0, 0.0, 0.0, 0.0, 0.0, 0.0, 0.0, 0.0, 0.0, 0.0, 0.0, 0.0, 0.0, 0.0, 0.0, 0.0, 0.0, 0.0, 0.0, 0.0, 0.0, 0.0, 0.0, 0.0, 0.0, 0.0, 0.0, 0.0, 0.0, 0.0, 0.0, 0.0, 0.0, 0.0, 0.0, 0.0, 0.0, 0.0, 0.0, 0.0, 0.0, 0.0, 0.0, 0.0, 0.0, 0.0, 0.0, 0.0, 0.0, 0.0, 0.0, 0.0, 0.0, 0.0, 0.0, 0.0, 0.0, 0.0, 0.0, 0.0, 0.0, 0.0, 0.0, 0.0, 0.0, 0.0, 0.0, 0.0, 0.0, 0.0, 0.0, 0.0, 0.0, 0.0, 0.0, 0.0, 0.0, 0.0, 0.0, 0.0, 0.0, 0.0, 0.0, 0.0, 0.0, 0.0, 0.0, 0.0, 0.0, 0.0, 0.0, 0.0, 0.0, 0.0, 0.0, 0.0, 0.0, 0.0, 0.0, 0.0, 0.0, 0.0, 0.0, 0.0, 0.0, 0.0, 0.0, 1.0], x=w72) -> (*(type *) &x=w67:dbl[])
      n18 = Type Cast(type=dbl[] [1.0, 1.0, 1.0, 1.0, 1.0, 1.0, 1.0, 1.0, 1.0, 1.0, 1.0, 1.0, 1.0, 1.0, 1.0, 1.0, 1.0, 1.0, 1.0, 1.0, 1.0, 1.0, 1.0, 1.0, 1.0, 1.0, 1.0, 1.0, 1.0, 1.0, 1.0, 1.0, 1.0, 1.0, 1.0, 1.0, 1.0, 1.0, 1.0, 1.0, 1.0, 1.0, 1.0, 1.0, 1.0, 1.0, 1.0, 1.0, 1.0, 1.0, 1.0, 1.0, 1.0, 1.0, 1.0, 1.0, 1.0, 1.0, 1.0, 1.0, 1.0, 1.0, 1.0, 1.0, 1.0, 1.0, 1.0, 1.0, 1.0, 1.0, 1.0, 1.0, 1.0, 1.0, 1.0, 1.0, 1.0, 1.0, 1.0, 1.0, 1.0, 1.0, 1.0, 1.0, 1.0, 1.0, 1.0, 1.0, 1.0, 1.0, 1.0, 1.0, 1.0, 1.0, 1.0, 1.0, 1.0, 1.0, 1.0, 1.0, 1.0, 1.0, 1.0, 1.0, 1.0, 1.0, 1.0, 1.0, 1.0, 1.0, 1.0, 1.0, 1.0, 1.0, 1.0, 1.0, 1.0, 1.0, 1.0, 1.0, 1.0, 1.0, 1.0, 1.0, 1.0, 1.0, 1.0, 1.0, 1.0, 1.0, 1.0, 1.0, 1.0, 1.0, 1.0, 1.0, 1.0, 1.0, 1.0, 1.0, 1.0, 1.0, 1.0, 1.0, 1.0, 1.0, 1.0, 1.0, 1.0, 1.0, 1.0, 1.0, 1.0, 1.0, 1.0, 1.0, 1.0, 1.0, 1.0, 1.0, 1.0, 1.0, 1.0, 1.0, 1.0, 1.0, 1.0, 1.0, 1.0, 1.0, 1.0, 1.0, 1.0, 1.0, 1.0, 1.0, 1.0, 1.0, 1.0, 1.0, 1.0, 1.0, 1.0, 1.0, 1.0, 1.0, 1.0, 1.0, 1.0, 1.0, 1.0, 1.0, 1.0, 1.0, 1.0, 1.0, 1.0, 1.0, 1.0, 1.0, 1.0, 1.0, 1.0, 1.0, 1.0, 1.0, 1.0, 1.0, 1.0, 1.0, 1.0, 1.0, 1.0, 1.0, 1.0, 1.0, 1.0, 1.0, 1.0, 1.0, 1.0, 1.0, 1.0, 1.0, 1.0, 1.0, 1.0, 1.0, 1.0, 1.0, 1.0, 1.0, 1.0, 1.0, 1.0, 1.0, 1.0, 1.0, 1.0, 1.0, 1.0, 1.0, 1.0, 1.0, 1.0, 1.0, 1.0, 1.0, 1.0, 1.0, 1.0, 1.0, 1.0, 1.0, 1.0, 1.0, 1.0, 1.0, 1.0, 1.0, 1.0, 1.0, 1.0, 1.0, 1.0, 1.0, 1.0, 1.0, 1.0, 1.0, 1.0, 1.0, 1.0, 1.0, 1.0, 1.0, 1.0, 1.0, 1.0, 1.0, 1.0, 1.0, 1.0, 1.0, 1.0, 1.0, 1.0, 1.0, 1.0, 1.0, 1.0, 1.0, 1.0, 1.0, 1.0, 1.0, 1.0, 1.0, 1.0, 1.0, 1.0, 1.0, 1.0, 1.0, 1.0, 1.0, 1.0, 1.0, 1.0, 1.0, 1.0, 1.0, 1.0, 1.0, 1.0, 1.0, 1.0, 1.0, 1.0, 1.0, 1.0, 1.0, 1.0, 1.0, 1.0, 1.0, 1.0, 1.0, 1.0, 1.0, 1.0, 1.0, 1.0, 1.0, 1.0, 1.0, 1.0, 1.0, 1.0, 1.0, 1.0, 1.0, 1.0, 1.0, 1.0, 1.0, 1.0, 1.0, 1.0, 1.0, 1.0, 1.0, 1.0, 1.0, 1.0, 1.0, 1.0, 1.0, 1.0, 1.0, 1.0, 1.0, 1.0, 1.0, 1.0, 1.0, 1.0, 1.0, 1.0, 1.0, 1.0, 1.0, 1.0, 1.0, 1.0, 1.0, 1.0, 1.0, 1.0, 1.0, 1.0, 1.0, 1.0, 1.0, 1.0, 1.0, 1.0, 1.0, 1.0, 1.0, 1.0, 1.0, 1.0, 1.0, 1.0, 1.0, 1.0, 1.0, 1.0, 1.0], x=w71) -> (*(type *) &x=w58:dbl[])
      n19 = Split 1D Array(array=w33, index=w87) -> (first subarray=→"XA":dbl[], second subarray=w36:dbl[])
      n20 = Split 1D Array(array=w67, index=w62) -> (first subarray=→"AD1":dbl[], second subarray=w59:dbl[])
      n21 = Split 1D Array(array=w58, index=w103) -> (first subarray=→"XB":dbl[], second subarray=w55:dbl[])
      n22 = Split 1D Array(array=w36, index=w112) -> (first subarray=→"YA":dbl[], second subarray=w79:dbl[])
      n23 = Split 1D Array(array=w59, index=w80) -> (first subarray=→"AD2":dbl[], second subarray=w66:dbl[])
      n24 = Split 1D Array(array=w55, index=w104) -> (first subarray=→"YB":dbl[], second subarray=w101:dbl[])
      n25 = Split 1D Array(array=w79, index=w88) -> (first subarray=→"FrequencyA":dbl[], second subarray=w39:dbl[])
      n26 = Split 1D Array(array=w66, index=w81) -> (first subarray=→"AD3":dbl[], second subarray=w65:dbl[])
      n27 = Split 1D Array(array=w101, index=w105) -> (first subarray=→"FrequencyB":dbl[], second subarray=w52:dbl[])
      n28 = Split 1D Array(array=w39, index=w111) -> (first subarray=→"NoiseA":dbl[], second subarray=w45:dbl[])
      n29 = Split 1D Array(array=w65, index=w82) -> (first subarray=→"AD4":dbl[])  [unwired: 1 out]
      n30 = Split 1D Array(array=w52, index=w110) -> (first subarray=→"NoiseB":dbl[], second subarray=w46:dbl[])
      n31 = Split 1D Array(array=w45, index=w91) -> (first subarray=→"Xh1A":dbl[], second subarray=w42:dbl[])
      n32 = Split 1D Array(array=w46, index=w106) -> (first subarray=→"Xh1B":dbl[], second subarray=w48:dbl[])
      n33 = Split 1D Array(array=w42, index=w92) -> (first subarray=→"Yh1A":dbl[], second subarray=w89:dbl[])
      n34 = Split 1D Array(array=w48, index=w107) -> (first subarray=→"Yh1B":dbl[], second subarray=w100:dbl[])
      n35 = Split 1D Array(array=w89, index=w93) -> (first subarray=→"Xh2A":dbl[], second subarray=w90:dbl[])
      n36 = Split 1D Array(array=w100, index=w108) -> (first subarray=→"Xh2B":dbl[], second subarray=w51:dbl[])
      n37 = Split 1D Array(array=w90, index=w94) -> (first subarray=→"Yh2A":dbl[])  [unwired: 1 out]
      n38 = Split 1D Array(array=w51, index=w109) -> (first subarray=→"Yh2B":dbl[])  [unwired: 1 out]
    }
    frame #2 {
      n39 = local read "FrequencyB"() -> (w168:dbl[])
      n40 = local read "FrequencyA"() -> (w160:dbl[])
      n41 = local read "FrequencyB"() -> (w128:dbl[])
      n42 = local read "NoiseB"() -> (w169:dbl[])
      n43 = local read "NoiseA"() -> (w161:dbl[])
      n44 = local read "NoiseB"() -> (w130:dbl[])
      n45 = local read "Xh1B"() -> (w170:dbl[])
      n46 = local read "Xh2B"() -> (w172:dbl[])
      n47 = local read "Xh1A"() -> (w162:dbl[])
      n48 = local read "Xh2A"() -> (w164:dbl[])
      n49 = local read "Yh1B"() -> (w171:dbl[])
      n50 = local read "Yh2B"() -> (w173:dbl[])
      n51 = local read "Yh1A"() -> (w163:dbl[])
      n52 = local read "Yh2A"() -> (w165:dbl[])
      n53 = local read "AD1"() -> (w174:dbl[])
      n54 = local read "AD2"() -> (w175:dbl[])
      n55 = local read "AD3"() -> (w176:dbl[])
      n56 = local read "AD4"() -> (w177:dbl[])
      n57 = local read "Xh1B"() -> (w131:dbl[])
      n58 = local read "Xh2B"() -> (w135:dbl[])
      n59 = local read "Xh2B"() -> (w133:dbl[])
      n60 = local read "Yh1B"() -> (w132:dbl[])
      n61 = local read "Yh2B"() -> (w134:dbl[])
      n62 = local read "XA"() -> (w158:dbl[])
      n63 = local read "YA"() -> (w159:dbl[])
      n64 = local read "XB"() -> (w166:dbl[])
      n65 = local read "YB"() -> (w167:dbl[])
      n66 = local read "XB"() -> (w127:dbl[])
      n67 = local read "YB"() -> (w129:dbl[])
      n68 = local read "AD1"() -> (w113:dbl[])
      n69 = local read "AD2"() -> (w114:dbl[])
      n70 = local read "AD3"() -> (w115:dbl[])
      n71 = local read "AD4"() -> (w116:dbl[])
      n72 = Bundle("AD1"=w113, "AD2"=w114, "AD3"=w115, "AD4"=w116) -> (→"输出簇ADC":T4)  [unwired: 1 in]
      n73 = Build Array(w158, w159, w160, w161, w162, w163, w164, w165, w166, w167, w168, w169, w170, w171, w172, w173, w174, w175, w176, w177) -> (→"总数组":dbl[][])
      n74 = Bundle("XB"=w127, "YB"=w129, "FrequencyB"=w128, "NoiseB"=w130, "Xh1B"=w131, "Yh1B"=w132, "Xh2B"=w135, "Yh2B"=w134, "Xh2B"=w133) -> (→"输出簇B":T2)  [unwired: 1 in]
      n75 = local read "FrequencyB"() -> (w147:dbl[])
      n76 = local read "FrequencyA"() -> (w143:dbl[])
      n77 = local read "NoiseB"() -> (w148:dbl[])
      n78 = local read "NoiseA"() -> (w142:dbl[])
      n79 = local read "Xh1B"() -> (w149:dbl[])
      n80 = local read "Xh2B"() -> (w151:dbl[])
      n81 = local read "Xh1A"() -> (w141:dbl[])
      n82 = local read "Xh2A"() -> (w139:dbl[])
      n83 = local read "Yh1B"() -> (w150:dbl[])
      n84 = local read "Yh2B"() -> (w152:dbl[])
      n85 = local read "Yh1A"() -> (w140:dbl[])
      n86 = local read "Yh2A"() -> (w138:dbl[])
      n87 = local read "AD4"() -> (w156:dbl[])
      n88 = local read "AD1"() -> (w153:dbl[])
      n89 = local read "AD2"() -> (w154:dbl[])
      n90 = local read "AD3"() -> (w155:dbl[])
      n91 = local read "XA"() -> (w137:dbl[])
      n92 = local read "YA"() -> (w144:dbl[])
      n93 = local read "XB"() -> (w145:dbl[])
      n94 = local read "YB"() -> (w146:dbl[])
      n95 = local read "FrequencyA"() -> (w119:dbl[])
      n96 = local read "NoiseA"() -> (w120:dbl[])
      n97 = local read "Xh1A"() -> (w121:dbl[])
      n98 = local read "Xh2A"() -> (w123:dbl[])
      n99 = local read "Yh1A"() -> (w122:dbl[])
      n100 = local read "Yh2A"() -> (w124:dbl[])
      n101 = local read "XA"() -> (w125:dbl[])
      n102 = local read "YA"() -> (w118:dbl[])
      n103 = Bundle("XA"=w137, "YA"=w144, "FrequencyA"=w143, "NoiseA"=w142, "Xh1A"=w141, "Yh1A"=w140, "Xh2A"=w139, "Yh2A"=w138, "XB"=w145, "YB"=w146, "FrequencyB"=w147, "NoiseB"=w148, "Xh1B"=w149, "Yh1B"=w150, "Xh2B"=w151, "Yh2B"=w152, "AD1"=w153, "AD2"=w154, "AD3"=w155, "AD4"=w156) -> (→"总输出簇":T1)  [unwired: 1 in]
      n104 = Bundle("XA"=w125, "YA"=w118, "FrequencyA"=w119, "NoiseA"=w120, "Xh1A"=w121, "Yh1A"=w122, "Xh2A"=w123, "Yh2A"=w124) -> (→"输出簇A":T3)  [unwired: 1 in]
    }
  }
